vi "Init Hardware.vi"(8 "error in (no error)":errorcluster, 11 "Temperature Controller Driver in":refnum<class "Temperature Controller Driver.lvclass">) -> (0 "error out":errorcluster, 3 "Temperature Controller Driver out":refnum<class "Temperature Controller Driver.lvclass">)   [LabVIEW 2016, in "Temperature Controller Driver.lvclass"]
uses:
  Temperature Controller Driver.lvclass
  C:/github/NHMFL_Core/Libraries/Instruments/Instrument Driver/Instrument Driver.lvclass
  Instrument Driver/Instrument Driver.lvclass/Instrument Driver.ctl
  Instrument Driver/Read Recorder name.vi
  Instrument Driver/Write Channel names.vi
  Instrument Driver/Write Channel units.vi
  Read T controller configuration.vi
  Simple VISA Reader/Simple VISA Reader Driver.lvclass
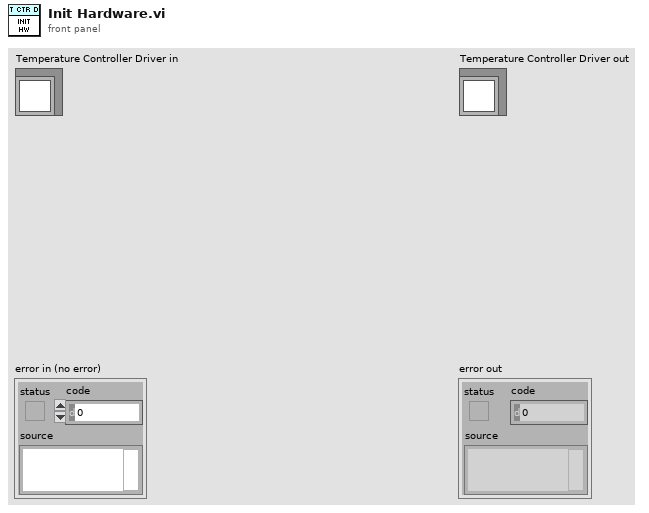
[diagram p1: front panel]
types:
  T1 = typedef "T controller configuration.ctl" = cluster{"Record Channels":string[], "Add raw signal":bool, "New set point":dbl}
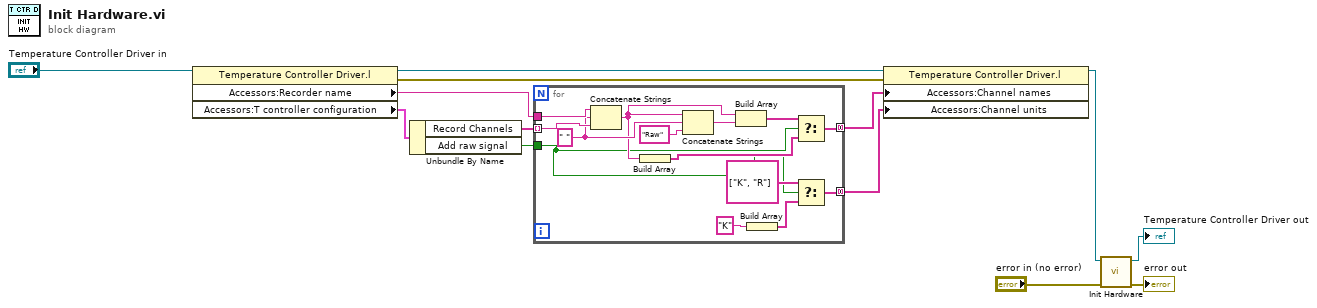
[diagram p0: block diagram]
diagram:
  n1 = property class="Temperature Controller Driver.l"(reference="Temperature Controller Driver in") -> (reference out=w8:refnum<class "Temperature Controller Driver.lvclass">, error out=w9:errorcluster, "Accessors:Recorder name"=w10:string, "Accessors:T controller configuration"=w5:T1)  [unwired: 1 in]
  n2 = Unbundle By Name(w5) -> ("Record Channels"=w4:string[], "Add raw signal"=w3:bool)
  n3 = for {
    tunnel: w4 -> [w26] mode=indexing
    tunnel: w3 -> [w14]
    tunnel: [w19] -> w2 mode=concatenating
    tunnel: [w15] -> w1 mode=concatenating
    tunnel: w10 -> [w27]
    w25 = " "
    n4 = Concatenate Strings(w27, w25, w26) -> (w23:string)
    n5 = Build Array(w23) -> (w20:string[])
    n6 = Concatenate Strings(w23, w25, "Raw" ("string")) -> (w22:string)
    n7 = Build Array(w23, w22) -> (w21:string[])
    n8 = Build Array("K") -> (w17:string[])
    n9 = Select(t=w21, s=w14, f=w20) -> (s? t:f=w19:string[])
    n10 = Select(t=string[] ["K", "R"], s=w14, f=w17) -> (s? t:f=w15:string[])
  }
  n11 = property class="Temperature Controller Driver.l"(reference=w8, error in=w9, "Accessors:Channel names"=w2, "Accessors:Channel units"=w1) -> (reference out=w6:refnum<class "Temperature Controller Driver.lvclass">)  [unwired: 1 out]
  n12 = call-parent "Init Hardware.vi"("error in (no error)"="error in (no error)", "Instrument Driver in"=w6) -> ("error out"=→"error out":errorcluster, "Instrument Driver out"=→"Temperature Controller Driver out":refnum<class "Temperature Controller Driver.lvclass">)  [unwired: 8 in]
